vi "Configure Event Enabled.vi"(8 "error in (no error)":errorcluster, 9 "Event Enabled (F: Disable)":bool, 10 "Event Action (0: Auxiliary Out)":i32(ring) items=["Auxiliary Out", "Print", "Save Image", "Save Waveform", "Service Request", "Stop Acquisition"], 11 "VISA resource name":refnum<visa-resource-name>) -> (0 "error out":errorcluster, 3 "VISA resource name out":refnum<visa-resource-name>)   [LabVIEW 2016, in "Tektronix DPO MSO 2000 4000 Series.lvlib"]
doc: "Configures the event action state.\n\n<B>Notes:</B>\nThis VI is available for MDO3000 Series only."
uses:
  Tektronix DPO MSO 2000 4000 Series.lvlib
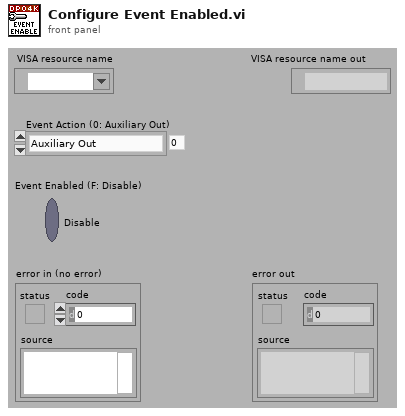
[diagram p1: front panel]
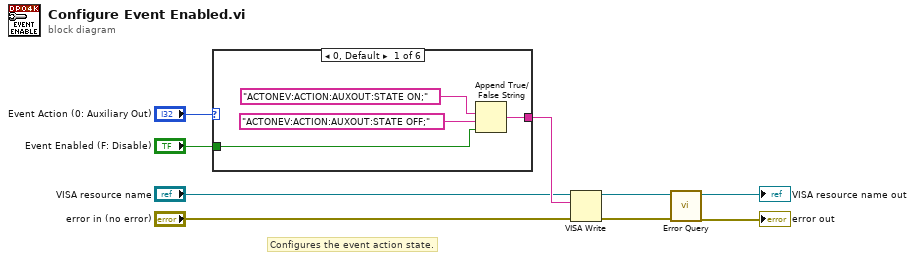
[diagram p0: block diagram]
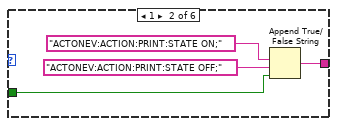
[diagram p2: hidden frame]
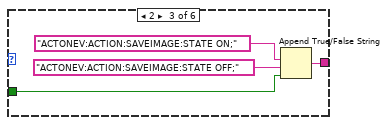
[diagram p3: hidden frame]
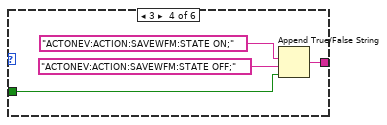
[diagram p4: hidden frame]
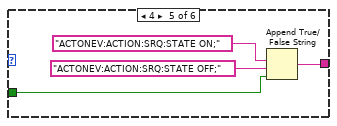
[diagram p5: hidden frame]
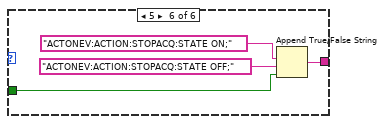
[diagram p6: hidden frame]
diagram:
  # "Configures the event action state."
  n1 = case shown="0, Default" "Event Action (0: Auxiliary Out)" {
    tunnel: [w11 w15 w19 w23 w27 w31] -> w3
    tunnel: "Event Enabled (F: Disable)" -> [w10 w14 w18 w22 w26 w30]
    frame 0, Default {
      n2 = Append True/False String(1:w10, 2:"ACTONEV:ACTION:AUXOUT:STATE OFF;", 3:"ACTONEV:ACTION:AUXOUT:STATE ON;") -> (0:w11:string)  [unwired: 1 in]
    }
    frame 1 {
      n3 = Append True/False String(1:w14, 2:"ACTONEV:ACTION:PRINT:STATE OFF;", 3:"ACTONEV:ACTION:PRINT:STATE ON;") -> (0:w15:string)  [unwired: 1 in]
    }
    frame 2 {
      n4 = Append True/False String(1:w18, 2:"ACTONEV:ACTION:SAVEIMAGE:STATE OFF;", 3:"ACTONEV:ACTION:SAVEIMAGE:STATE ON;") -> (0:w19:string)  [unwired: 1 in]
    }
    frame 3 {
      n5 = Append True/False String(1:w22, 2:"ACTONEV:ACTION:SAVEWFM:STATE OFF;", 3:"ACTONEV:ACTION:SAVEWFM:STATE ON;") -> (0:w23:string)  [unwired: 1 in]
    }
    frame 4 {
      n6 = Append True/False String(1:w26, 2:"ACTONEV:ACTION:SRQ:STATE OFF;", 3:"ACTONEV:ACTION:SRQ:STATE ON;") -> (0:w27:string)  [unwired: 1 in]
    }
    frame 5 {
      n7 = Append True/False String(1:w30, 2:"ACTONEV:ACTION:STOPACQ:STATE OFF;", 3:"ACTONEV:ACTION:STOPACQ:STATE ON;") -> (0:w31:string)  [unwired: 1 in]
    }
  }
  n8 = VISA Write(VISA resource name="VISA resource name", write buffer=w3, error in (no error)="error in (no error)") -> (VISA resource name out=w8:refnum<visa-resource-name>, error out=w7:errorcluster)  [unwired: 1 out]
  n9 = call "Error Query.vi"("error in (no error)"=w7, "VISA resource name"=w8) -> ("error out"=→"error out":errorcluster, "VISA resource name out"=→"VISA resource name out":refnum<visa-resource-name>)  [unwired: 6 in, 2 out]
